vi "get info constant.vi"() -> (0 "set":set{string}(c389), 1 "String":string)   [LabVIEW 2023, in "Publisher Subscriber.lvlib"]
uses:
  <userlib>/_Publisher Subscriber/Publisher Subscriber.lvlib
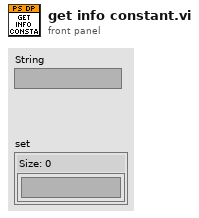
[diagram p1: front panel]
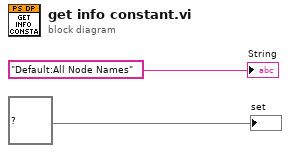
[diagram p0: block diagram]
diagram:
  "set" <- set{string} {} ("set")
  "String" <- "Default:All Node Names"
